vi "Import Transactions from File.vi"(8 "error in (no error)":errorcluster) -> (0 "error out":errorcluster, 3 "Importing Statement":refnum<class "TransactionList.lvclass">)   [LabVIEW 2018]
uses:
  classes/Statement/TransactionList.lvclass
  <vilib>/Utility/sysdir.llb/System Directory Type.ctl
  classes/Banking Statement/Banking Transactions.lvclass
  C:/GitRepos/Filthy-Lucre-Budgetizer/source/support/classes/Statement/TransactionList.lvclass
  classes/Credit Statement/Credit Transactions.lvclass
  classes/Banking Record/Banking Transaction.lvclass
  C:/GitRepos/Filthy-Lucre-Budgetizer/source/support/classes/Transaction/Transaction.lvclass
  classes/Credit Record/Credit Transaction.lvclass
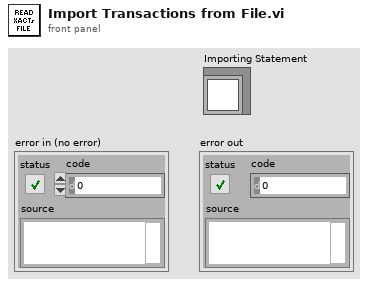
[diagram p1: front panel]
types:
  T1 = typedef "System Directory Type.ctl" = i32
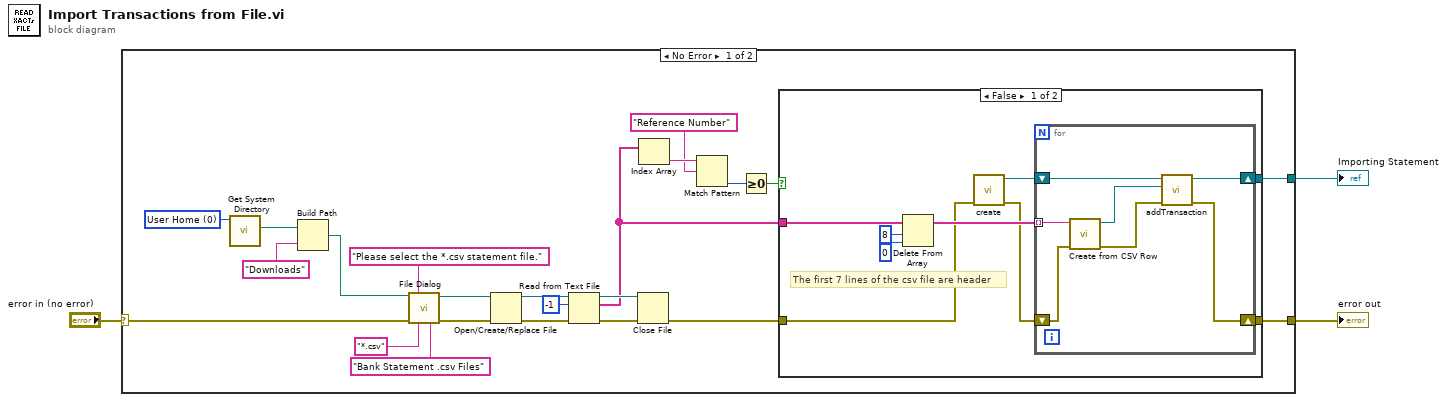
[diagram p0: block diagram]
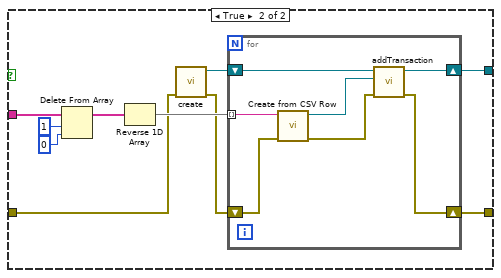
[diagram p2: hidden frame]
diagram:
  n1 = case shown="No Error" "error in (no error)" {
    selector: "error in (no error)" -> [w12 w60]
    tunnel: [w10 w60] -> w3
    tunnel: [w9 _] -> w1
    frame No Error {
      w16 = T1 0 items=["User Home"=0, "User Desktop"=1, "User Documents"=2, "User Application Data"=3, "User Preferences"=4, "User Temporary"=5, "Public Documents"=6, "Public Application Data"=7, "Public Preferences"=8, "Public Cache"=13, "System Core Libraries"=9, "System Installed Libraries"=10, "Application Files"=11, "Boot Volume Root"=12] ("system directory type")
      n2 = call <vilib>:"Get System Directory.vi"("system directory type"=w16) -> ("system directory"=w15:path)  [unwired: 10 in]
      n3 = Build Path(base path=w15, name or relative path="Downloads") -> (appended path=w13:path)
      n4 = call "File Dialog"("start path"=w13, "prompt"="Please select the *.csv statement file.", "error in"=w12, "pattern (all files)"="*.csv", "pattern label"="Bank Statement .csv Files") -> ("selected path"=w18:path, "error out"=w17:errorcluster)  [unwired: 2 in, 7 out]
      n5 = Open/Create/Replace File(file path (use dialog)=w18, error in=w17) -> (refnum out=w23:refnum<file>, error out=w22:errorcluster)  [unwired: 5 out]
      n6 = Read from Text File(file (use dialog)=w23, count=-1, error in=w22) -> (refnum out=w20:refnum<file>, text=w8:string[], error out=w21:errorcluster)  [unwired: 2 out]
      n7 = Close File(refnum=w20, error in=w21) -> (error out=w11:errorcluster)  [unwired: 1 out]
      n8 = Index Array(array=w8) -> (element=w7:string)  [unwired: 1 in]
      n9 = Match Pattern(string=w7, regular expression="Reference Number") -> (offset past match=w5:i32)  [unwired: 1 in, 3 out]
      n10 = Greater Or Equal To 0?(x=w5) -> (x >= 0?=w4:bool)
      n11 = case shown="False" w4 {
        tunnel: w11 -> [w28 w44]
        tunnel: [w31 w46] -> w10
        tunnel: [w30 w47] -> w9
        tunnel: w8 -> [w32 w48]
        frame False {
          # "The first 7 lines of the csv file are header"
          n12 = Delete From Array(array=w32, length=8, index=0) -> (array with subset deleted=w33:string[])  [unwired: 1 out]
          n13 = call "create.vi"("error in (no error)"=w28) -> ("error out"=w27:errorcluster, "Banking Transactions out"=w29:refnum<class "Banking Transactions.lvclass">)  [unwired: 9 in]
          n14 = for {
            tunnel: w33 -> [w42] mode=indexing
            shift-right: [w36] -> w31
            shift-left: w27 -> [w41]
            shift-right: [w39] -> w30
            shift-left: w29 -> [w40]
            n15 = call "Create from CSV Row.vi"("error in (no error)"=w41, "CSV Row"=w42) -> ("error out"=w37:errorcluster, "Banking Record"=w38:refnum<class "Banking Transaction.lvclass">)  [unwired: 8 in]
            n16 = call "addTransaction.vi"("error in (no error)"=w37, "Transaction.lvclass"=w38, "TransactionList in"=w40) -> ("error out"=w36:errorcluster, "TransactionList out"=w39:refnum<class "Banking Transactions.lvclass">)  [unwired: 7 in]
          }
        }
        frame True {
          n17 = Delete From Array(array=w48, length=1, index=0) -> (array with subset deleted=w50:string[])  [unwired: 1 out]
          n18 = Reverse 1D Array(array=w50) -> (reversed array=w49:string[])
          n19 = call "create.vi"("error in (no error)"=w44) -> ("error out"=w43:errorcluster, "Credit Transactions out"=w45:refnum<class "Credit Transactions.lvclass">)  [unwired: 9 in]
          n20 = for {
            shift-right: [w54] -> w46
            shift-left: w43 -> [w58]
            tunnel: w49 -> [w59] mode=indexing
            shift-right: [w53] -> w47
            shift-left: w45 -> [w57]
            n21 = call "Create from CSV Row.vi"("error in (no error)"=w58, "CSV Row"=w59) -> ("error out"=w55:errorcluster, "Credit Record out"=w56:refnum<class "Credit Transaction.lvclass">)  [unwired: 8 in]
            n22 = call "addTransaction.vi"("error in (no error)"=w55, "Transaction.lvclass"=w56, "TransactionList in"=w57) -> ("error out"=w54:errorcluster, "TransactionList out"=w53:refnum<class "Credit Transactions.lvclass">)  [unwired: 7 in]
          }
        }
      }
    }
    frame Error {
    }
  }
  "error out" <- w3
  "Importing Statement" <- w1
